vi "AIT 1553 - License Status.vi"(11 "error in (no error)":errorcluster) -> (4 "license file info out":T1, 6 "license status":T2(ring), 15 "error out":errorcluster)   [LabVIEW 2015, in "AIT 1553 Custom Device.lvlib"]
uses:
  AIT 1553 Custom Device.lvlib
  <vilib>/AddonLicensing/SoftwareKeyLicensingProvider.llb/_SK_LicenseFileInfo.ctl
panel:
  in  "license file info":T1
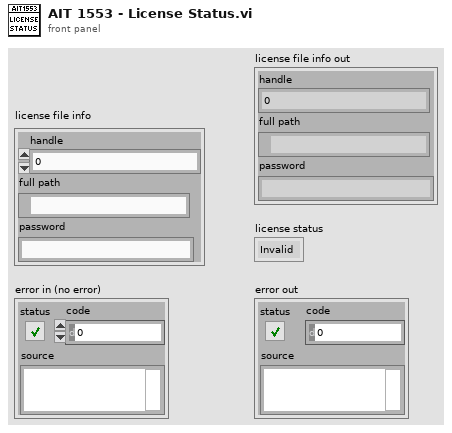
[diagram p1: front panel]
types:
  T1 = typedef "NI_LV2PLicAPI.lvlib/_SK_LicenseFileInfo.ctl" = cluster{"handle":i32, "full path":path, "password":string}
  T2 = enum16{"Invalid", "Expired", "Evaluation", "Activated"}
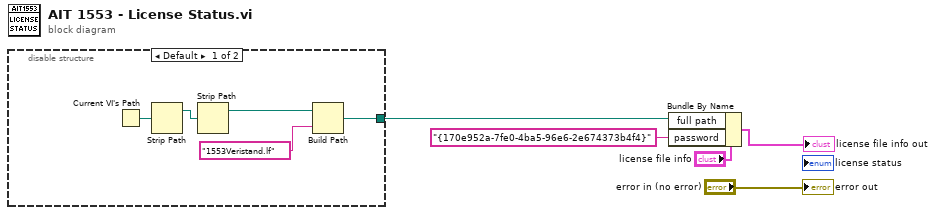
[diagram p0: block diagram]
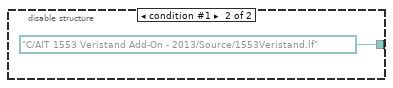
[diagram p2: hidden frame]
diagram:
  n1 = disable-structure shown="Default" {
    disable-tunnel: [w8 path "C:/AIT 1553 Veristand Add-On - 2013/Source/1553Veristand.lf" ("appended path")] -> w3
    frame condition #0 (active) {
      n2 = Current VI's Path() -> (path=w6:path)
      n3 = Strip Path(path=w6) -> (stripped path=w9:path)  [unwired: 1 out]
      n4 = Strip Path(path=w9) -> (stripped path=w10:path)  [unwired: 1 out]
      n5 = Build Path(base path=w10, name or relative path="1553Veristand.lf") -> (appended path=w8:path)
    }
    frame condition #1 {
    }
  }
  n6 = Bundle By Name(cluster="license file info", "full path"=w3, "password"="{170e952a-7fe0-4ba5-96e6-2e674373b4f4}") -> (→"license file info out":T1)
  "error out" <- "error in (no error)"
